vi "convMto10 (SubVI).vi"(10 "old base":i32=16, 11 "value":i32[](array[numeric])) -> (3 "converted value":i32=2147483647)   [LabVIEW 2017]
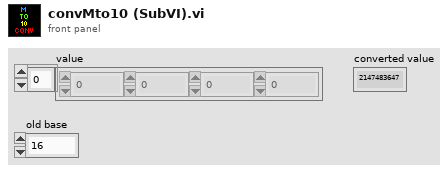
[diagram p1: front panel]
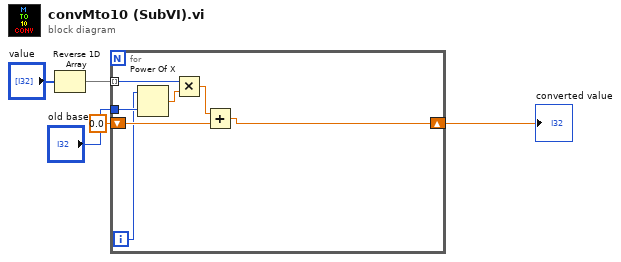
[diagram p0: block diagram]
diagram:
  n1 = Reverse 1D Array(array="value") -> (reversed array=w2:i32[])
  n2 = for {
    shift-right: [w12] -> w3
    shift-left: 0.0 -> [w11]
    tunnel: "old base" -> [w10]
    tunnel: w2 -> [w9] mode=indexing
    i -> [w6]
    n3 = Power Of X(1:w10, 2:w6) -> (0:w8:dbl)
    n4 = Multiply(x=w9, y=w8) -> (x*y=w7:dbl)
    n5 = Add(x=w7, y=w11) -> (x+y=w12:dbl)
  }
  "converted value" <- w3
